vi "shelving_time.vi"(2 "in t/f":bool) -> (0 "out t/f":bool)   [LabVIEW 2012]
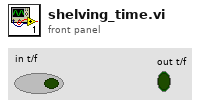
[diagram p1: front panel]
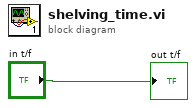
[diagram p0: block diagram]
diagram:
  "out t/f" <- "in t/f"
